vi "Draw Text at Point with Pixel Font.vi"(8 "string":string="Hello", 10 "origin":cluster{"x":i16, "y":i16}, 11 "picture":picture) -> (3 "picture out":picture)   [LabVIEW 2021, in "Picture Pixel Fonts.lvlib"]
uses:
  <vilib>/LabVIEW Icon API/Pixel Fonts/Picture Pixel Fonts.lvlib
  <vilib>/LabVIEW Icon API/Pixel Fonts/Pixel Font/Pixel Font.lvlib
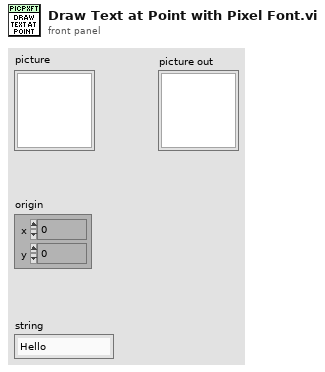
[diagram p1: front panel]
types:
  T1 = typedef "imagedata.ctl" = cluster{"image type":i32, "image depth":i32, "image":u8[], "mask":u8[], "colors":u32[], "Rectangle":cluster{"left":i16, "top":i16, "right":i16, "bottom":i16}}
  T2 = cluster{"left":i16, "top":i16, "right":i16, "bottom":i16}
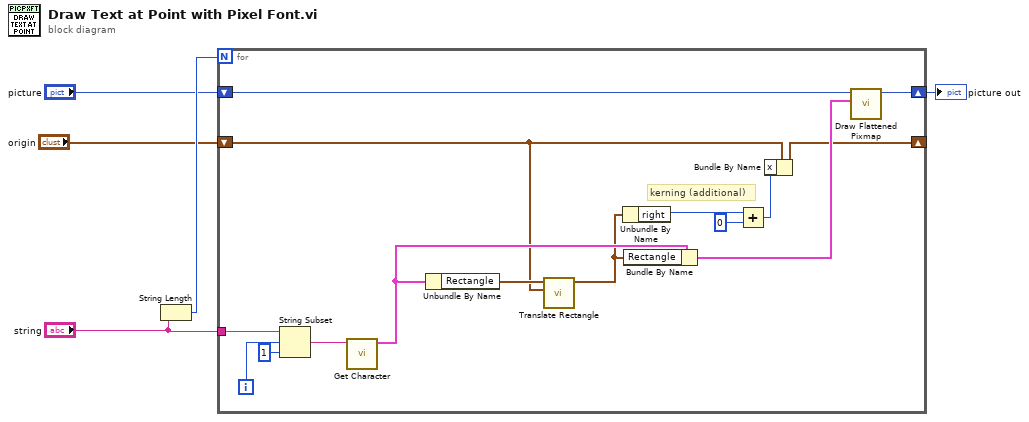
[diagram p0: block diagram]
diagram:
  n1 = String Length(string="string") -> (length=w4:i32)
  n2 = for {
    N: w4 -> [_]
    tunnel: "string" -> [w19]
    shift-right: [w6] -> _
    shift-left: "origin" -> [w8]
    shift-right: [w15] -> w2
    shift-left: "picture" -> [w16]
    i -> [w17]
    # "kerning (additional)"
    n3 = String Subset(string=w19, offset (0)=w17, length (rest)=1 ("length (rest)")) -> (substring=w18:string)
    n4 = call <vilib>:"Get Character.vi"("string"=w18) -> ("image data"=w14:T1)  [unwired: 10 in]
    n5 = Unbundle By Name(w14) -> ("Rectangle"=w9:T2)
    n6 = call <vilib>:"Translate Rectangle.vi"("offset"=w8, "Rectangle in"=w9) -> ("Rectangle out"=w11:T2)  [unwired: 9 in]
    n7 = Unbundle By Name(w11) -> ("right"=w10:i16)
    n8 = Bundle By Name(cluster=w14, "Rectangle"=w11) -> (w13:T1)
    n9 = Add(x=w10, y=i16 0) -> (x+y=w7:i16)
    n10 = Bundle By Name(cluster=w8, "x"=w7) -> (w6:cluster{"x":i16, "y":i16})
    n11 = call <vilib>:"Draw Flattened Pixmap.vi"("image data"=w13, "picture"=w16) -> ("new picture"=w15:picture)  [unwired: 7 in]
  }
  "picture out" <- w2
